vi "MFLI--reader--V2.vi"() -> ()   [LabVIEW 2017]
uses:
  publisher action.ctl
  MFLI frontend action.ctl
panel:
  in  "all":enum32{"all", "other"}(tab)
  out "read Voltage (V)":cdb=7.620420552454007e-07+0.00015686579971617868i format="%#10_10f"
  in  "read !":bool
  out "read Voltage X (V)":dbl=-9.280888050611169e-06 format="%#11_11f"
  out "read Voltage Y (V)":dbl=-2.2786646865421625e-05 format="%#11_11f"
  in  "delay-read (msec)":i64=50
  out "read freq (Hz)":dbl=30901.670598808552 format="%-#.3f"
  in  "MFLI Address":string="DEV3523"
  in  "Exit !":bool
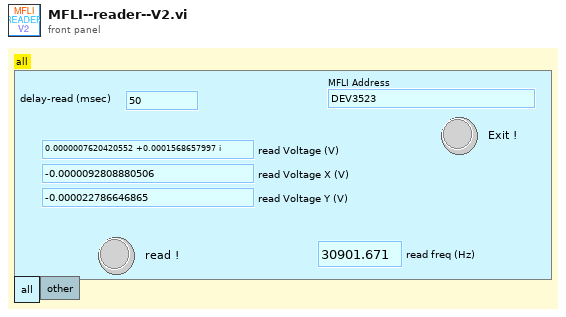
[diagram p1: front panel]
types:
  T1 = typedef "MFLI frontend action.ctl" = enum16{"read", "writeread", "open", "close", "write"}
  T2 = typedef "publisher action.ctl" = enum16{"set", "get"}
  T3 = typedef "Zurich Instruments LabOne.lvlib/ziTypeHandle.ctl" = cluster{"handleValid":bool, "Conn":u64, "Path Prefix":string, "Handle":u64, "Connected":bool, "Clockbase(s)":dbl}
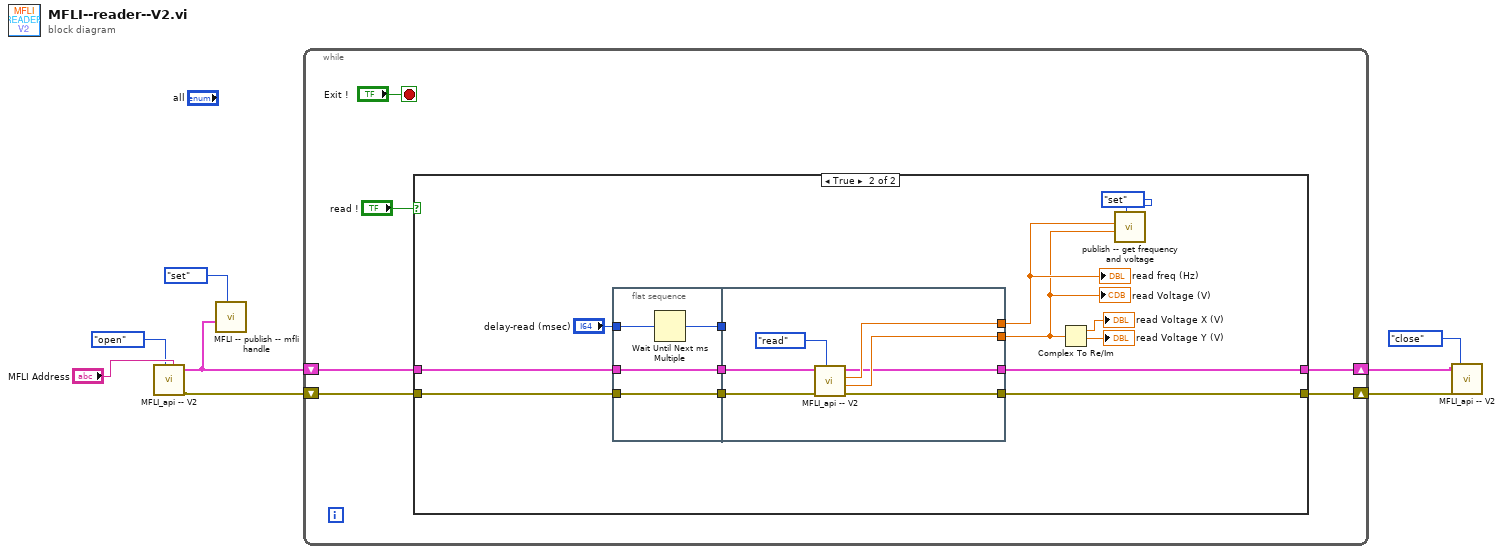
[diagram p0: block diagram]
diagram:
  n1 = call "MFLI_api -- V2.vi"("MFLI Address"="MFLI Address", "MFLI frontend action"=MFLI_frontend_action."open") -> ("Error Out"=w6:errorcluster, "Handle Out"=w5:T3)  [unwired: 6 in, 2 out]
  n2 = call "MFLI -- publish -- mfli handle.vi"("publisher action"=publisher_action."set", "Handle IN"=w5) -> ()  [unwired: 9 in, 1 out]
  n3 = while {
    shift-right: [w12] -> w2
    shift-left: w6 -> [w13]
    shift-right: [w9] -> w3
    shift-left: w5 -> [w10]
    stop <- "Exit !" stop-if-true
    n4 = case shown="True" "read !" {
      tunnel: w13 -> [w16 w24]
      tunnel: [w16 w23] -> w12
      tunnel: w10 -> [w15 w19]
      tunnel: [w15 w17] -> w9
      frame False {
      }
      frame True {
        n5 = flat-sequence {
          tunnel: [w33] -> w29
          tunnel: "delay-read (msec)" -> [w32]
          tunnel: [w31] -> w25
          tunnel: w24 -> [w31]
          tunnel: w19 -> [w30]
          tunnel: [w30] -> w18
          tunnel: w29 -> [_]
          tunnel: [w38] -> w20
          tunnel: [w37] -> w21
          tunnel: w25 -> [w40]
          tunnel: [w39] -> w23
          tunnel: w18 -> [w36]
          tunnel: [w35] -> w17
          frame #0 {
            n6 = Wait Until Next ms Multiple(millisecond multiple=w32) -> (millisecond timer value=w33:u32)
          }
          frame #1 {
            n7 = call "MFLI_api -- V2.vi"("MFLI frontend action"=MFLI_frontend_action."read", "Error In"=w40, "Handle In"=w36) -> ("Error Out"=w39:errorcluster, "z out (V)"=w38:cdb, "Freq out (Hz)"=w37:dbl, "Handle Out"=w35:T3)  [unwired: 5 in]
          }
        }
        n8 = Complex To Re/Im(x + iy=w20) -> (x=→"read Voltage X (V)":dbl, y=→"read Voltage Y (V)":dbl)
        n9 = call "publish -- get frequency and voltage.vi"("publisher action"=publisher_action."set", "Voltage IN (V)"=w20, "freq IN (Hz)"=w21) -> ()  [unwired: 7 in, 2 out]
        "read Voltage (V)" <- w20
        "read freq (Hz)" <- w21
      }
    }
  }
  n10 = call "MFLI_api -- V2.vi"("MFLI frontend action"=MFLI_frontend_action."close", "Error In"=w2, "Handle In"=w3) -> ()  [unwired: 5 in, 4 out]
